vi "CALW Batch Command.vi"() -> ()   [LabVIEW 2018]
panel:
  out "S4ICS cmd":string
  out "LOG time":timestamp format="%<%H:%M:%S%3u\n%Y/%m/%d>T"
  in  "mechanism name":string="CALW" caption="(WPROT, CALW, ...)"
  in  "allin":T1={"s4icsIP"="localhost", "s4icsPort"=54165, "mech name"="", "cmd"=[], "log"=refnum} {"s4icsPort" min=1025 step=1}
  in  "stop":bool
  # "S4ICS Batch Command"
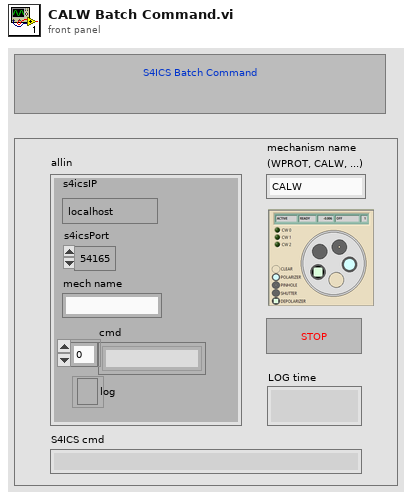
[diagram p1: front panel]
types:
  T1 = cluster{"s4icsIP":string, "s4icsPort":u16, "mech name":string, "cmd":string[], "log":refnum<file>}
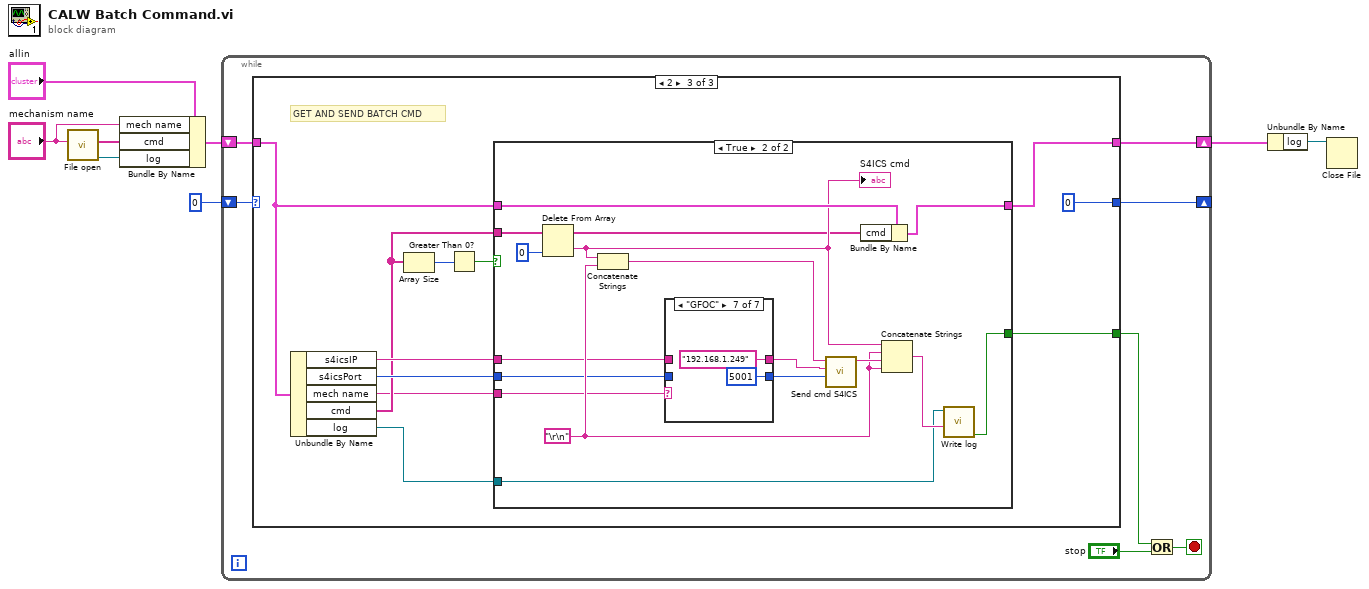
[diagram p0: block diagram]
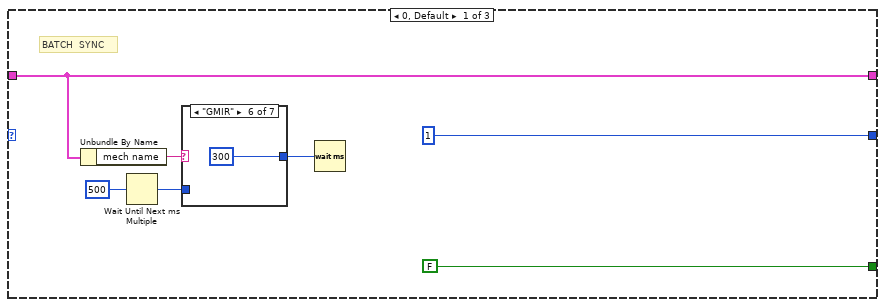
[diagram p2: hidden frame]
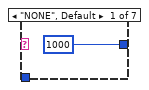
[diagram p3: hidden frame]
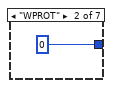
[diagram p4: hidden frame]
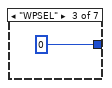
[diagram p5: hidden frame]
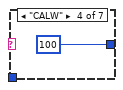
[diagram p6: hidden frame]
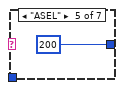
[diagram p7: hidden frame]
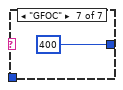
[diagram p8: hidden frame]
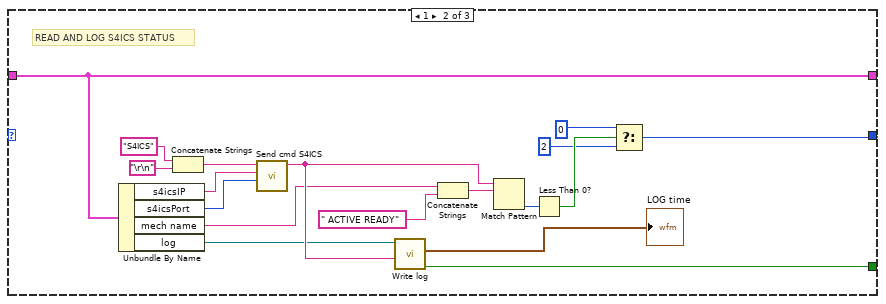
[diagram p9: hidden frame]
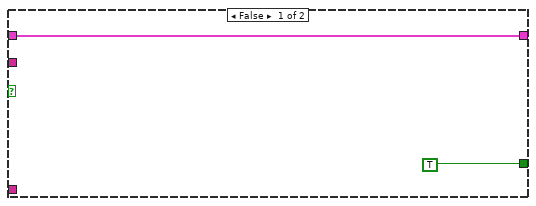
[diagram p10: hidden frame]
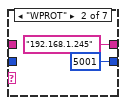
[diagram p12: hidden frame]
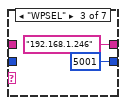
[diagram p13: hidden frame]
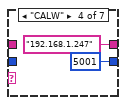
[diagram p14: hidden frame]
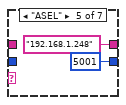
[diagram p15: hidden frame]
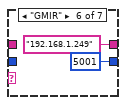
[diagram p16: hidden frame]
diagram:
  n1 = call "File open.vi"("mech name"="mechanism name") -> ("log"=w5:refnum<file>, "cmd"=w4:string[])  [unwired: 9 in]
  n2 = Bundle By Name(cluster="allin", "mech name"="mechanism name", "cmd"=w4, "log"=w5) -> (w6:T1)
  n3 = while {
    shift-right: [w14] -> _
    shift-left: u8 0 -> [w15]
    shift-right: [w12] -> w2
    shift-left: w6 -> [w13]
    stop <- w10 stop-if-true
    n4 = case shown="2" w15 {
      tunnel: [u8 1 ("x+1") w38 u8 0 ("x+1")] -> w14
      tunnel: w13 -> [w19 w40 w54]
      tunnel: [w19 w40 w51] -> w12
      tunnel: [FALSE w35 w53] -> w9
      frame 0, Default {
        # "BATCH  SYNC"
        n5 = Unbundle By Name(w19) -> ("mech name"=w18:string)
        n6 = Wait Until Next ms Multiple(millisecond multiple=u32 500) -> (millisecond timer value=w16:u32)
        n7 = case shown="\"GMIR\"" w18 {
          tunnel: [u32 1000 ("millisecond multiple") u32 0 ("millisecond multiple") u32 0 ("millisecond multiple") u32 100 ("millisecond multiple") u32 200 ("millisecond multiple") u32 300 ("millisecond multiple") u32 400 ("millisecond multiple")] -> w22
          tunnel: w16 -> [_ _ _ _ _ _ _]
          frame "NONE", Default {
          }
          frame "WPROT" {
          }
          frame "WPSEL" {
          }
          frame "CALW" {
          }
          frame "ASEL" {
          }
          frame "GMIR" {
          }
          frame "GFOC" {
          }
        }
        n8 = Wait (ms)(milliseconds to wait=w22) -> ()  [unwired: 1 out]
      }
      frame 1 {
        # "READ AND LOG S4ICS STATUS"
        n9 = Unbundle By Name(w40) -> ("s4icsIP"=w45:string, "s4icsPort"=w44:u16, "mech name"=w32:string, "log"=w34:refnum<file>)
        n10 = Concatenate Strings("S4ICS", "\r\n") -> (w43:string)
        n11 = call "Send cmd S4ICS.vi"("port"=w44, "address"=w45, "data in"=w43) -> ("data out"=w36:string)  [unwired: 7 in, 1 out]
        n12 = call "Write log.vi"("text"=w36, "log file"=w34) -> ("status"=w35:bool, "current time"=→"LOG time":timestamp)  [unwired: 8 in]
        n13 = Concatenate Strings(w32, " ACTIVE READY") -> (w33:string)
        n14 = Match Pattern(string=w36, regular expression=w33) -> (offset past match=w42:i32)  [unwired: 1 in, 3 out]
        n15 = Less Than 0?(x=w42) -> (x < 0?=w39:bool)
        n16 = Select(t=u8 0 ("f"), s=w39, f=u8 2) -> (s? t:f=w38:u8)
      }
      frame 2 {
        # "GET AND SEND BATCH CMD"
        n17 = Unbundle By Name(w54) -> ("s4icsIP"=w58:string, "s4icsPort"=w57:u16, "mech name"=w49:string, "cmd"=w50:string[], "log"=w48:refnum<file>)
        n18 = Array Size(array=w50) -> (size(s)=w56:i32)
        n19 = Greater Than 0?(x=w56) -> (x > 0?=w55:bool)
        n20 = case shown="True" w55 {
          tunnel: w58 -> [_ w64]
          tunnel: w57 -> [_ w63]
          tunnel: w50 -> [_ w77]
          tunnel: w54 -> [w60 w76]
          tunnel: [w60 w75] -> w51
          tunnel: [TRUE w69] -> w53
          tunnel: w49 -> [_ w65]
          tunnel: w48 -> [_ w66]
          frame False {
          }
          frame True {
            w67 = "\r\n"
            n21 = Delete From Array(array=w77, index=0) -> (deleted portion=w72:string, array with subset deleted=w70:string[])  [unwired: 1 in]
            "S4ICS cmd" <- w72
            n22 = Concatenate Strings(w72, w67) -> (w74:string)
            n23 = case shown="\"GFOC\"" w65 {
              tunnel: w64 -> [w79 _ _ _ _ _ _]
              tunnel: w63 -> [w78 _ _ _ _ _ _]
              tunnel: [w79 "192.168.1.245" ("s4icsIP") "192.168.1.246" ("s4icsIP") "192.168.1.247" ("s4icsIP") "192.168.1.248" ("s4icsIP") "192.168.1.249" ("s4icsIP") "192.168.1.249" ("s4icsIP")] -> w62
              tunnel: [w78 u16 5001 ("s4icsPort") u16 5001 ("s4icsPort") u16 5001 ("s4icsPort") u16 5001 ("s4icsPort") u16 5001 ("s4icsPort") u16 5001 ("s4icsPort")] -> w61
              frame "NONE", Default {
              }
              frame "WPROT" {
              }
              frame "WPSEL" {
              }
              frame "CALW" {
              }
              frame "ASEL" {
              }
              frame "GMIR" {
              }
              frame "GFOC" {
              }
            }
            n24 = call "Send cmd S4ICS.vi"("port"=w61, "address"=w62, "data in"=w74) -> ("data out"=w73:string)  [unwired: 7 in, 1 out]
            n25 = Bundle By Name(cluster=w76, "cmd"=w70) -> (w75:T1)
            n26 = Concatenate Strings(w72, w67, w73, w67) -> (w71:string)
            n27 = call "Write log.vi"("text"=w71, "log file"=w66) -> ("status"=w69:bool)  [unwired: 8 in, 1 out]
          }
        }
      }
    }
    n28 = Or(x=w9, y="stop") -> (x .or. y?=w10:bool)
  }
  n29 = Unbundle By Name(w2) -> ("log"=w1:refnum<file>)
  n30 = Close File(refnum=w1) -> ()  [unwired: 1 in, 2 out]
